vi "brc_daq_set_parameters.vi"(0 "sample_rate":dbl, 1 "coupling_mode":i32, 2 "current_mA":dbl, 5 "error in (no error)":errorcluster, 6 "mHandle":i32) -> (19 "error out":errorcluster)   [LabVIEW 2019, in "BRC-DAQ.lvlib"]
uses:
  BRC-DAQ.lvlib
panel:
  out "return_value":i32
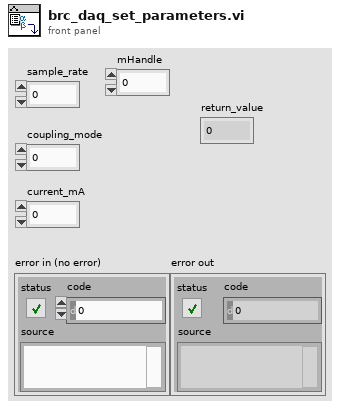
[diagram p1: front panel]
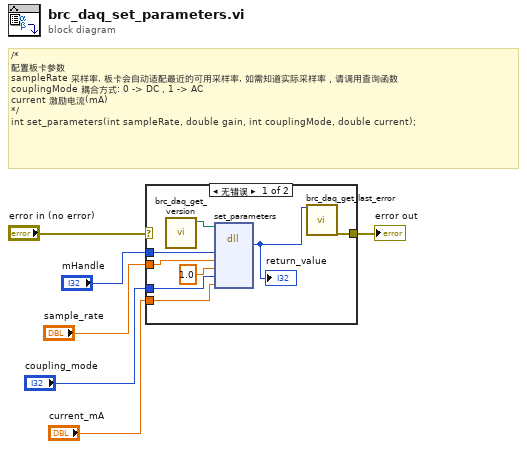
[diagram p0: block diagram]
diagram:
  # "/*\n配置板卡参数\nsampleRate 采样率, 板卡会自动适配最近的可用采样率, 如需知道实际采样率，请调用查询函数\ncouplingMode 耦合方式: 0 -> DC , 1 -> AC\ncurrent 激励电流(mA)\n*/\nint set_parameters(int sampleRate, double gain, int couplingMode, double current);"
  n1 = case shown="无错误" "error in (no error)" {
    selector: "error in (no error)" -> [_ w15]
    tunnel: "sample_rate" -> [w14 _]
    tunnel: "coupling_mode" -> [w13 _]
    tunnel: "current_mA" -> [w12 _]
    tunnel: [w10 w15] -> w3
    tunnel: "mHandle" -> [w8 _]
    frame No Error {
      n2 = call "brc_daq_get_version.vi"() -> ("dll path"=w7:path)  [unwired: 11 in]
      n3 = dll-call lib="E:/01 BRC project/04BRC-daq/04 Drive/BRC-DAQ/DAQ/DLL/32/brc_daq_sdk.dll" fn="set_parameters"(path in=w7, "mHandle"=w8, "sampleRate"=w14, "gain"=1.0, "couplingMode"=w13, "current"=w12) -> ("return type"=w11:i32)  [unwired: 7 in, 2 out]
      "return_value" <- w11
      n4 = call "brc_daq_get_last_error.vi"("return_value"=w11) -> ("error out"=w10:errorcluster)  [unwired: 18 in]
    }
    frame Error {
    }
  }
  "error out" <- w3
